vi "Microscope.TestLauncher.vi"() -> ()   [LabVIEW 2013]
doc: "JKI State Machine Objects (SMO) 1.0.0.5\nJKI - JKI\nCopyright (c) 2016, JKI"
uses:
  <vilib>/JKI/JKI SMO/SMO/SMO.lvclass
  Microscope.lvclass
  <vilib>/JKI/JKI SMO/SMO/Typedefs/SMOState --Enum.ctl
  <vilib>/Utility/error.llb/DialogType.ctl
  XYStage/Typedefs/(real)Coords--Cluster.ctl
  XYStage/XYStage.lvclass
  XYStage/Typedefs/PublicEvents--XYStage.UpdatedNamedPosition.ctl
  XYStage/Typedefs/PublicEvents--Cluster.ctl
  Camera/Typedefs/PublicEvents--Cluster.ctl
  Camera/Camera.lvclass
panel:
  in  "Settings":bool
  in  "Stop 2":bool caption="Stop"
  out "Camera model":string caption="CAMERA MODEL:"
  out "Image":picture
  out "Motion in Progress":bool
  out "Initialized":bool
  out "Well":string
  out "Position":string
  out "XYStage model":string caption="XY STAGE MODEL:"
  in  "Save Info":enum32{"Well Position", "Coordinates"}(radio)
  out "image path":path
  in  "Experiment":string
  in  "Save Images to Disk":bool
  out "Stage":picture
  in  "CaptureImmediately":bool
  in  "Coords":T1
  out "State":T2
  in  "CaptureAtPosition":bool
  out "error out":errorcluster
  # "MICROSCOPE CONTROLLER"
  # "Current Status"
  # "XY STAGE CONTROLLER"
  # "Current Address"
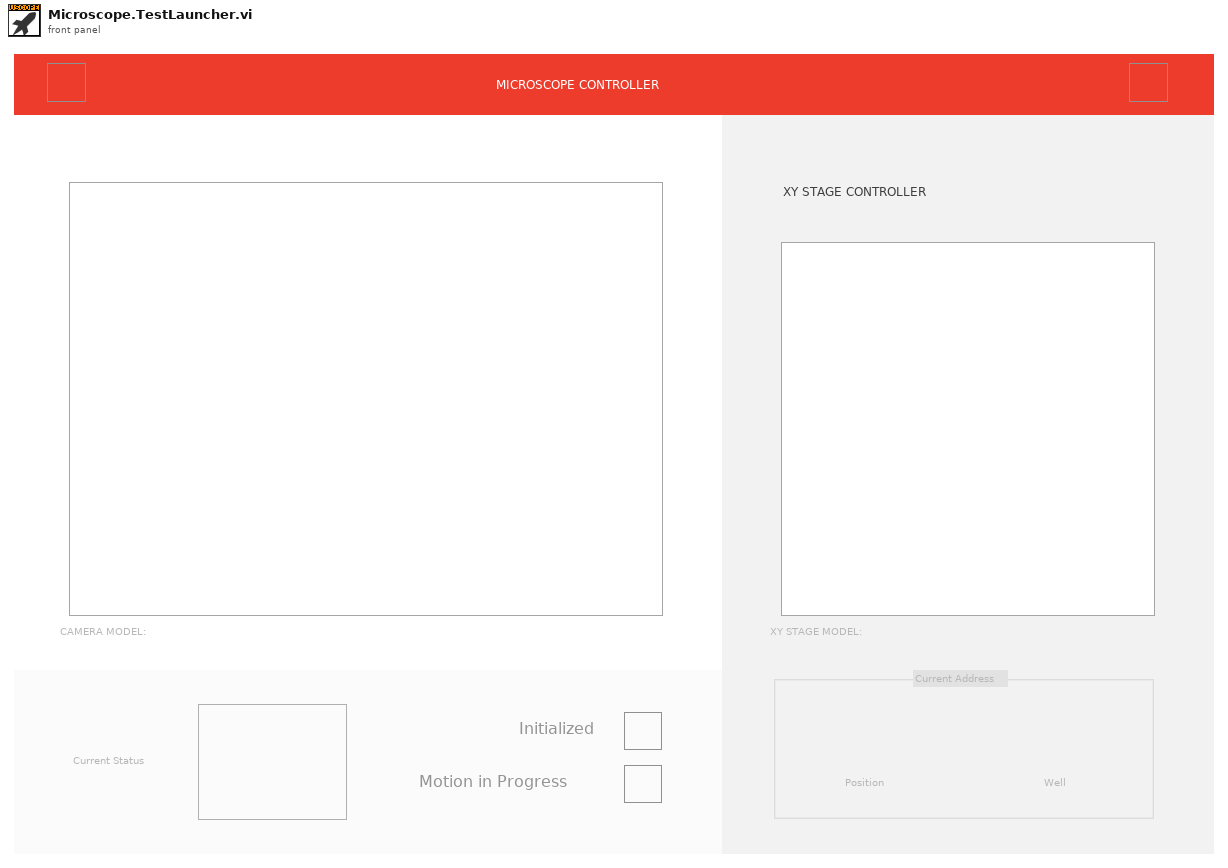
[diagram p1: front panel]
types:
  T1 = typedef "XYStage.lvclass/(real)Coords--Cluster.ctl" = cluster{"X":dbl, "Y":dbl}
  T2 = typedef "SMO.lvclass/SMOState --Enum.ctl" = enum16{"unknown", "Created", "Started", "Stopped"}
  T3 = cluster{"left":i16, "top":i16, "right":i16, "bottom":i16}
  T4 = typedef "Camera.lvclass/PublicEvents--Cluster.ctl" = cluster{"NewImage":refnum<user-event>, "ImageSaved":refnum<user-event>}
  T5 = typedef "XYStage.lvclass/PublicEvents--Cluster.ctl" = cluster{"MoveComplete":refnum<user-event>, "NewPosition":refnum<user-event>, "UpdatedNamedPosition":refnum<user-event>, "MoveStarted":refnum<user-event>}
  T6 = typedef "Microscope.lvclass/PublicEvents--Cluster.ctl" = cluster{"Value Changed":refnum<user-event>, "Initialized":refnum<user-event>}
  T7 = typedef "SMO.lvclass/Public Events.ctl" = cluster{"Error":refnum<user-event>, "State":refnum<user-event>}
  T8 = cluster{"Event Registration Refnum":refnum<event-registration>}
  T9 = typedef "imagedata.ctl" = cluster{"image type":i32, "image depth":i32, "image":u8[], "mask":u8[], "colors":u32[], "Rectangle":cluster{"left":i16, "top":i16, "right":i16, "bottom":i16}}
  T10 = typedef "LVMouseTypeDef.ctl" = cluster{"Mouse Position":cluster{"X":i32, "Y":i32}, "Mouse Modifiers":cluster{"Button Down":bool, "Shift Mod":bool, "Menu Mod":bool, "Option Mod":bool}}
  T11 = typedef "DialogType.ctl" = u16
  T12 = typedef "Microscope.lvclass/PublicEvents--Microscope.Initialized.ctl" = bool
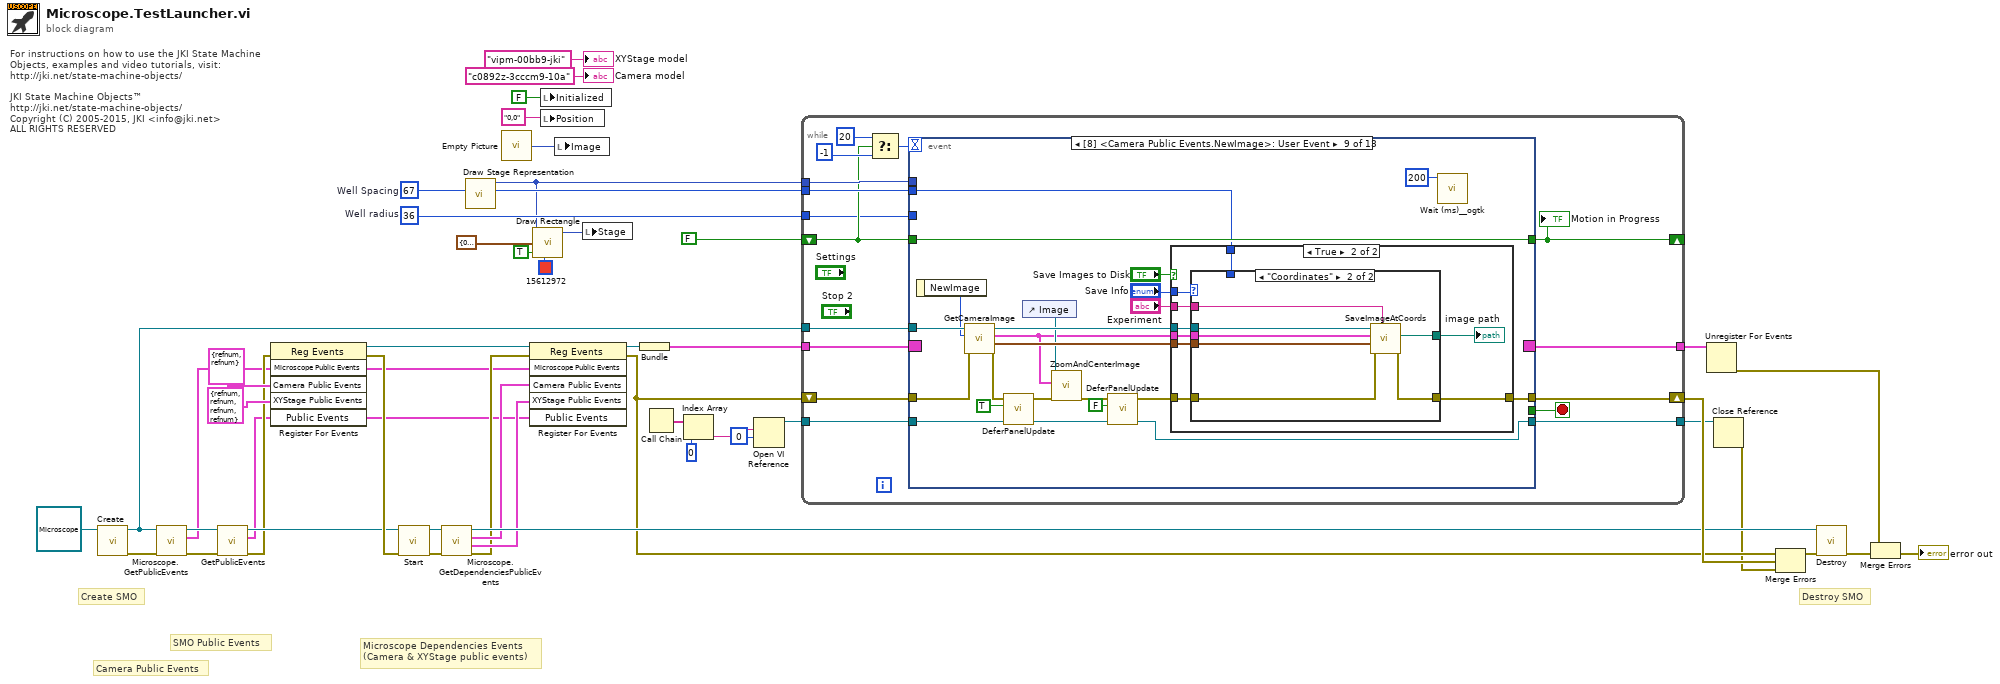
[diagram p0: block diagram]
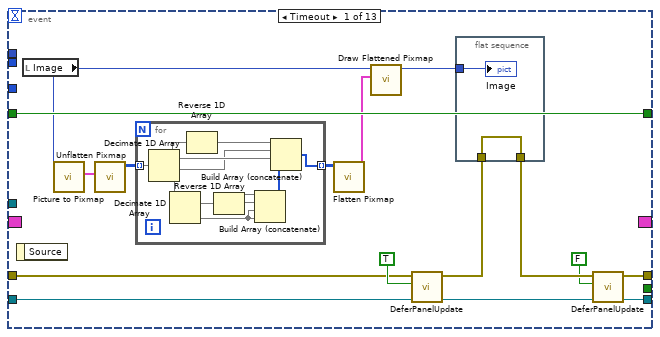
[diagram p2: hidden frame]
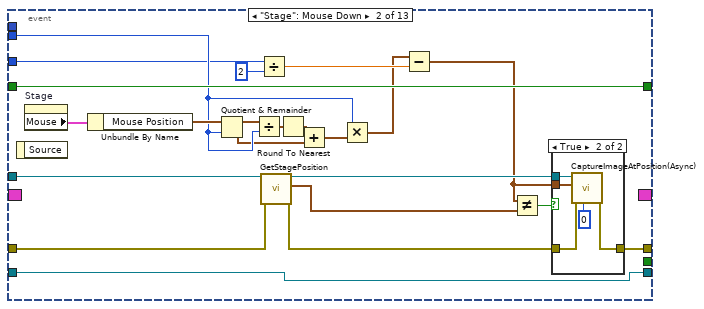
[diagram p3: hidden frame]
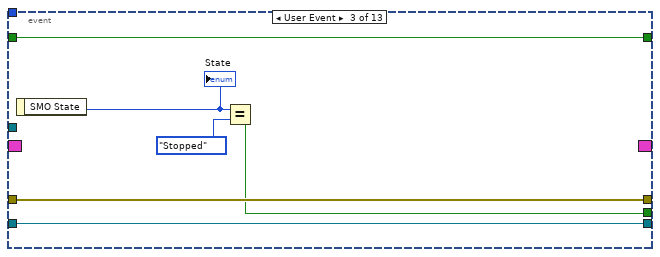
[diagram p5: hidden frame]
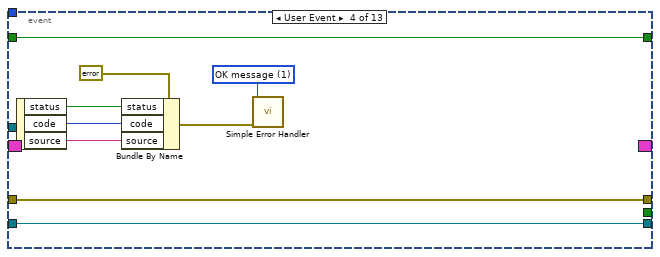
[diagram p6: hidden frame]
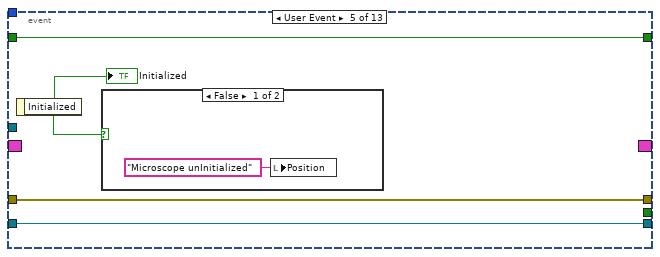
[diagram p7: hidden frame]
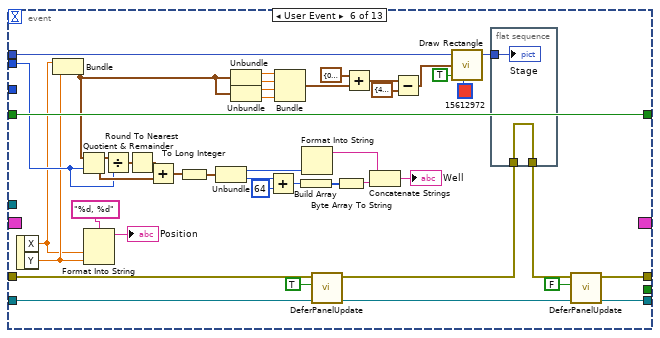
[diagram p9: hidden frame]
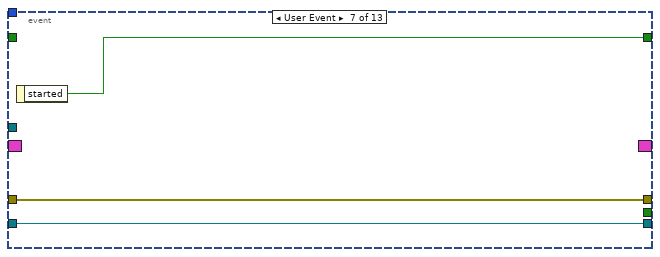
[diagram p10: hidden frame]
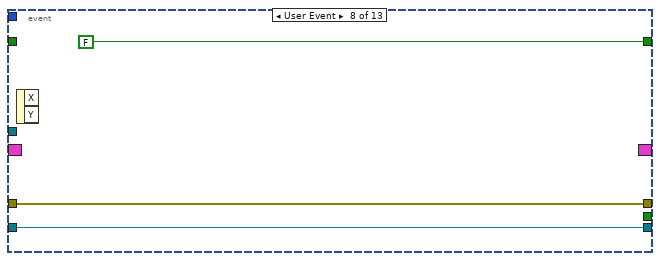
[diagram p11: hidden frame]
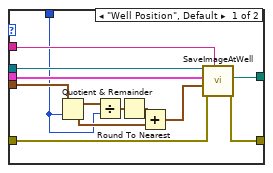
[diagram p13: hidden frame]
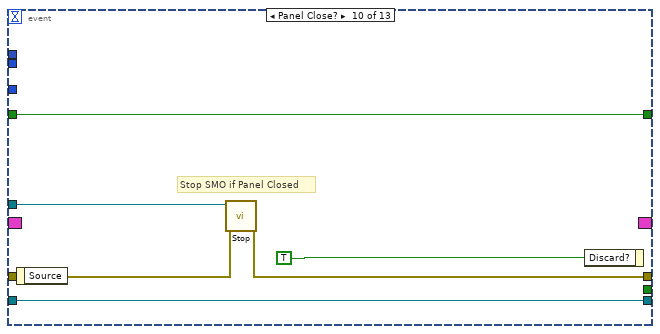
[diagram p14: hidden frame]
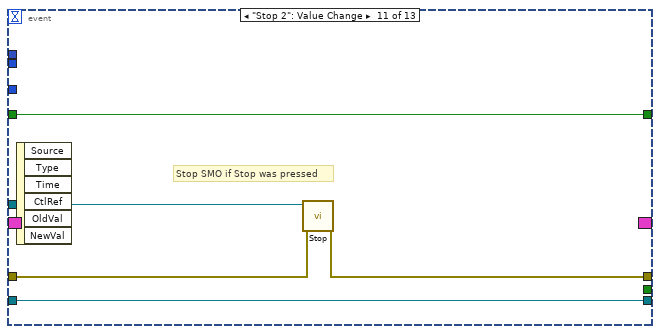
[diagram p15: hidden frame]
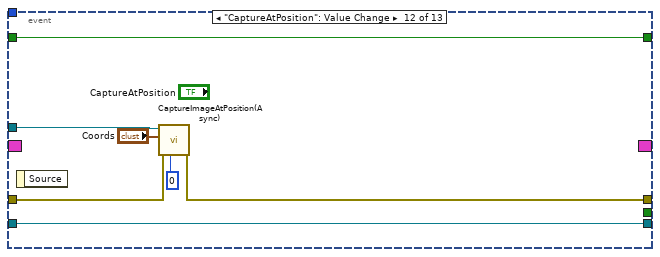
[diagram p16: hidden frame]
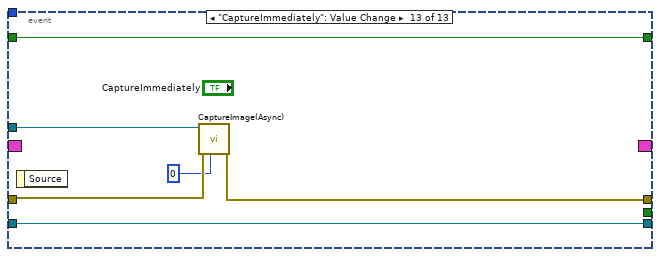
[diagram p17: hidden frame]
diagram:
  w15 = i16 36  # Well radius
  w3 = i16 67  # Well Spacing
  # "Microscope Dependencies Events\n(Camera & XYStage public events)"
  # "SMO Public Events"
  # "For instructions on how to use the JKI State Machine Objects, examples and video tutorials, visit:\nhttp://jki.net/state-machine-objects/\n\nJKI State Machine Objects™\nhttp://jki.net/state-machine-objects/\nCopyright (C) 2005-2015, JKI <info@jki.net>\nALL RIGHTS RESERVED"
  # "Camera Public Events"
  # "Destroy SMO"
  # "Create SMO"
  n1 = call <vilib>:"Create.vi"("SMO"=refnum<class "Microscope.lvclass"> refnum ("SMO.Template.lvclass")) -> ("error out"=w38:errorcluster, "SMO out"=w39:refnum<class "Microscope.lvclass">)  [unwired: 8 in, 1 out]
  n2 = call "Microscope.GetPublicEvents.vi"("error in (no error)"=w38, "Microscope"=w39) -> ("error out"=w41:errorcluster, "Microscope Public Events"=w19:T6, "Microscope out"=w42:refnum<class "Microscope.lvclass">)  [unwired: 7 in]
  n3 = call <vilib>:"GetPublicEvents.vi"("error in (no error)"=w41, "SMO"=w42) -> ("error out"=w29:errorcluster, "Public Events"=w18:T7, "SMO out"=w30:refnum<class "Microscope.lvclass">)  [unwired: 7 in]
  n4 = register-events(error in=w29, w19, T4 {"NewImage"=refnum, "ImageSaved"=refnum} ("Camera Public Events"), T5 {"MoveComplete"=refnum, "NewPosition"=refnum, "UpdatedNamedPosition"=refnum, "MoveStarted"=refnum} ("XYStage Public Events"), w18) -> (reference out=w25:refnum<event-registration>, error out=w37:errorcluster)  [unwired: 1 in]
  n5 = call <vilib>:"Start.vi"("error in (no error)"=w37, "SMO"=w30) -> ("error out"=w26:errorcluster, "SMO out"=w28:refnum<class "Microscope.lvclass">)  [unwired: 8 in]
  n6 = call "Microscope.GetDependenciesPublicEvents.vi"("error in (no error)"=w26, "Microscope"=w28) -> ("error out"=w21:errorcluster, "XYStage Public Events"=w22:T5, "Camera Public Events"=w23:T4, "Microscope out"=w27:refnum<class "Microscope.lvclass">)  [unwired: 6 in]
  n7 = call "Draw Stage Representation.vi"("Well Spacing"=w3) -> ("Well Spacing out"=w2:i16, "new picture"=w1:picture)  [unwired: 9 in]
  n8 = call "Empty Picture"() -> ("empty picture"=w33:picture)
  n9 = register-events(reference=w25, error in=w21, w19, w23, w22, w18) -> (reference out=w24:refnum<event-registration>, error out=w20:errorcluster)
  n10 = call <vilib>:"Draw Rectangle.vi"("picture"=w1, "rect"=T3 {"left"=0, "top"=0, "right"=6, "bottom"=6}, "fill?(F)"=TRUE, "color(black)"=u32 15612972) -> ("new picture"=w11:picture)  [unwired: 5 in]
  n11 = local write "Initialized"(FALSE ("Initialized")) -> ()
  n12 = local write "Position"("0,0" ("Position")) -> ()
  n13 = local write "Image"(w33) -> ()
  n14 = local write "Stage"(w11) -> ()
  n15 = Bundle("Event Registration Refnum"=w24) -> (w48:T8)  [unwired: 1 in]
  n16 = Call Chain() -> (call chain=w7:string[])
  n17 = Index Array(array=w7, index=0 ("Index")) -> (element=w9:string)
  n18 = Open VI Reference(vi path=w9, options=0) -> (vi reference=w6:refnum<vi>)  [unwired: 4 in, 1 out]
  n19 = while {
    shift-right: [w64] -> w47
    shift-left: w20 -> [w63]
    tunnel: w48 -> [w62]
    tunnel: [w61] -> w49
    tunnel: w39 -> [w60]
    shift-right: [w59] -> _
    shift-left: FALSE -> [w54]
    tunnel: w1 -> [w58]
    tunnel: w2 -> [w57]
    tunnel: w15 -> [w52]
    tunnel: w6 -> [w51]
    tunnel: [w50] -> w5
    stop <- w65 stop-if-true
    n20 = Select(t=20, s=w54, f=-1) -> (s? t:f=w55:i32)
    n21 = event shown="[8] <Camera Public Events.NewImage>: User Event" {
      selector: w62 -> [_ _ _ _ _ _ _ _ _ _ _ _ _]
      dyn-events: [_ _ _ _ _ _ _ _ _ _ _ _ _] -> w61
      timeout: w55 -> [_ _ _ _ _ _ _ _ _ _ _ _ _]
      tunnel: [_ _ w125 _ _ _ _ _ _ _ _ _ _] -> w65
      tunnel: w60 -> [_ w106 _ _ _ _ _ _ w216 w252 w257 w263 w270]
      tunnel: [w73 w114 w128 w137 w141 w145 w190 w193 w211 w251 w256 w259 w268] -> w64
      tunnel: w63 -> [w76 w104 w128 w137 w141 w150 w190 w193 w214 w250 w255 w261 w269]
      tunnel: [w81 w116 w124 w136 w139 w183 w189 FALSE w213 w248 w254 w264 w266] -> w59
      tunnel: w54 -> [w81 w116 w124 w136 w139 w183 _ _ w213 w248 w254 w264 w266]
      tunnel: w58 -> [_ _ _ _ _ w168 _ _ _ _ _ _ _]
      tunnel: w57 -> [_ w112 _ _ _ w178 _ _ w206 _ _ _ _]
      tunnel: w52 -> [_ w101 _ _ _ _ _ _ _ _ _ _ _]
      tunnel: w51 -> [w74 w95 w123 w129 w138 w149 w188 w191 w202 w247 w253 w258 w265]
      tunnel: [w72 w95 w123 w129 w138 w143 w188 w191 w198 w247 w253 w258 w265] -> w50
      event Timeout {
        n22 = event-data() -> ()  [unwired: 1 in, 1 out]
        n23 = local read "Image"() -> (w68:picture)
        n24 = call <vilib>:"Picture to Pixmap.vi"("picture"=w68) -> ("image data"=w80:T9)  [unwired: 9 in, 1 out]
        n25 = call <vilib>:"Unflatten Pixmap.vi"("image data"=w80) -> ("24-bit pixmap"=w79:u32[][])  [unwired: 4 in, 6 out]
        n26 = for {
          tunnel: w79 -> [w94] mode=indexing
          tunnel: [w90] -> w78 mode=indexing
          n27 = Decimate 1D Array(w94) -> (w93:u32[], w92:u32[], w91:u32[], w89:u32[])
          n28 = Decimate 1D Array(w89) -> (w88:u32[], w85:u32[])  [unwired: 2 out]
          n29 = Reverse 1D Array(array=w93) -> (reversed array=w87:u32[])
          n30 = Reverse 1D Array(array=w88) -> (reversed array=w86:u32[])
          n31 = Build Array (concatenate)(w86, w86, w85, w85) -> (w84:u32[])
          n32 = Build Array (concatenate)(w87, w91, w92, w84) -> (w90:u32[])
        }
        n33 = call <vilib>:"Flatten Pixmap.vi"("24-bit pixmap"=w78) -> ("image data"=w67:T9)  [unwired: 10 in]
        n34 = call <vilib>:"Draw Flattened Pixmap.vi"("image data"=w67, "picture"=w68) -> ("new picture"=w66:picture)  [unwired: 7 in]
        n35 = call "DeferPanelUpdate.vi"("VI in"=w74, "defer panel updates"=TRUE, "error in (no error)"=w76) -> ("VI out"=w71:refnum<vi>, "error out"=w75:errorcluster)  [unwired: 7 in]
        n36 = flat-sequence {
          tunnel: w66 -> [w83]
          tunnel: [w82] -> w70
          tunnel: w75 -> [w82]
          frame #0 {
            "Image" <- w83
          }
        }
        n37 = call "DeferPanelUpdate.vi"("VI in"=w71, "defer panel updates"=FALSE, "error in (no error)"=w70) -> ("VI out"=w72:refnum<vi>, "error out"=w73:errorcluster)  [unwired: 7 in]
      }
      event "Stage": Mouse Down {
        n38 = event-data() -> ()  [unwired: 1 in, 1 out]
        n39 = property on="Stage" class="Pict"() -> ("Mouse"=w115:T10)  [unwired: 2 in, 2 out]
        n40 = Unbundle By Name(w115) -> ("Mouse Position"=w113:cluster{"X":i32, "Y":i32})
        n41 = Quotient & Remainder(x=w113, y=w112) -> (x-y*floor(x/y)=w110:cluster{"X":i32, "Y":i32}, floor(x/y)=w108:cluster{"X":i32, "Y":i32})
        n42 = Divide(x=w110, y=w112) -> (x/y=w111:cluster{"X":dbl, "Y":dbl})
        n43 = Divide(x=w101, y=i16 2) -> (x/y=w99:dbl)
        n44 = call "GetStagePosition.vi"("error in (no error)"=w104, "Microscope"=w106) -> ("error out"=w103:errorcluster, "Coords"=w102:T1, "Microscope out"=w105:refnum<class "Microscope.lvclass">)  [unwired: 7 in]
        n45 = Round To Nearest(number=w111) -> (nearest integer value=w109:cluster{"X":dbl, "Y":dbl})
        n46 = Add(x=w109, y=w108) -> (x+y=w98:cluster{"X":dbl, "Y":dbl})
        n47 = Multiply(x=w112, y=w98) -> (x*y=w97:cluster{"X":dbl, "Y":dbl})
        n48 = Subtract(x=w97, y=w99) -> (x-y=w96:cluster{"X":dbl, "Y":dbl})
        n49 = Not Equal?(x=w96, y=w102) -> (x != y?=w107:bool)
        n50 = case shown="True" w107 {
          tunnel: w105 -> [_ w122]
          tunnel: w103 -> [w117 w120]
          tunnel: [w117 w119] -> w114
          tunnel: w96 -> [_ w121]
          frame False {
          }
          frame True {
            n51 = call "CaptureImageAtPosition(Async).vi"("timeout in ms (5000)"=0, "error in (no error)"=w120, "Coords"=w121, "Microscope"=w122) -> ("error out"=w119:errorcluster)  [unwired: 5 in, 2 out]
          }
        }
      }
      event User Event {
        n52 = event-data() -> ("SMO State"=w127:T2)  [unwired: 1 in]
        "State" <- w127
        n53 = Equal?(x=w127, y=SMOState_--Enum."Stopped") -> (x = y?=w125:bool)
      }
      event User Event {
        w133 = T11 1 items=["no dialog", "OK message", "continue or stop message", "OK message + warnings", "continue/stop + warnings"] ("type of dialog (OK msg:1)")
        n54 = event-data() -> ("status"=w132:bool, "code"=w131:i32, "source"=w130:string)  [unwired: 1 in]
        n55 = Bundle By Name(cluster=errorcluster {"status"=FALSE, "code"=0, "source"=""} ("error out"), "status"=w132, "code"=w131, "source"=w130) -> (w134:errorcluster)
        n56 = call <vilib>:"Simple Error Handler.vi"("type of dialog (OK msg:1)"=w133, "error in (no error)"=w134) -> ()  [unwired: 3 in, 5 out]
      }
      event User Event {
        n57 = event-data() -> ("Initialized"=w140:T12)  [unwired: 1 in]
        "Initialized" <- w140
        n58 = case shown="False" w140 {
          frame False {
            n59 = local write "Position"("Microscope unInitialized" ("Position")) -> ()
          }
          frame True {
          }
        }
      }
      event User Event {
        n60 = event-data() -> ("X"=w161:dbl, "Y"=w162:dbl)  [unwired: 1 in]
        n61 = Bundle("X"=w161, "Y"=w162) -> (w159:cluster{"X":dbl, "Y":dbl})  [unwired: 1 in]
        n62 = Quotient & Remainder(x=w159, y=w178) -> (x-y*floor(x/y)=w181:cluster{"X":dbl, "Y":dbl}, floor(x/y)=w179:cluster{"X":dbl, "Y":dbl})
        n63 = Format Into String(format string="%d, %d", w161, w162) -> (resulting string=→"Position":string)  [unwired: 2 in, 1 out]
        n64 = Divide(x=w181, y=w178) -> (x/y=w182:cluster{"X":dbl, "Y":dbl})
        n65 = Round To Nearest(number=w182) -> (nearest integer value=w180:cluster{"X":dbl, "Y":dbl})
        n66 = Add(x=w180, y=w179) -> (x+y=w177:cluster{"X":dbl, "Y":dbl})
        n67 = To Long Integer(number=w177) -> (32bit integer=w176:cluster{"X":i32, "Y":i32})
        n68 = Unbundle(w176) -> ("X"=w171:i32, "Y"=w175:i32)
        n69 = Unbundle(w159) -> ("X"=w158:dbl, "Y"=w157:dbl)
        n70 = Unbundle(w159) -> ("X"=w160:dbl, "Y"=w156:dbl)
        n71 = Add(x=w175, y=64 ("x")) -> (x+y=w173:i32)
        n72 = Bundle("X"=w158, "Y"=w157, "X"=w160, "Y"=w156) -> (w164:cluster{"X":dbl, "Y":dbl, "X":dbl, "Y":dbl})  [unwired: 1 in]
        n73 = Build Array(w173) -> (w174:i32[])
        n74 = Format Into String(w171) -> (resulting string=w152:string)  [unwired: 3 in, 1 out]
        n75 = call "DeferPanelUpdate.vi"("VI in"=w149, "defer panel updates"=TRUE, "error in (no error)"=w150) -> ("VI out"=w144:refnum<vi>, "error out"=w148:errorcluster)  [unwired: 7 in]
        n76 = Byte Array To String(unsigned byte array=w174) -> (string=w170:string)
        n77 = Add(x=T3 {"left"=0, "top"=0, "right"=13, "bottom"=13} ("rect"), y=w164) -> (x+y=w155:cluster{dbl, dbl, dbl, dbl})
        n78 = Concatenate Strings(w152, w170) -> (→"Well":string)
        n79 = Subtract(x=w155, y=cluster{dbl, dbl, dbl, dbl} {4.0, 3.0, 4.0, 3.0}) -> (x-y=w154:cluster{dbl, dbl, dbl, dbl})
        n80 = call <vilib>:"Draw Rectangle.vi"("picture"=w168, "rect"=w154, "fill?(F)"=TRUE, "color(black)"=u32 15612972) -> ("new picture"=w165:picture)  [unwired: 5 in]
        n81 = flat-sequence {
          tunnel: w165 -> [w187]
          tunnel: [w186] -> w146
          tunnel: w148 -> [w186]
          frame #0 {
            "Stage" <- w187
          }
        }
        n82 = call "DeferPanelUpdate.vi"("VI in"=w144, "defer panel updates"=FALSE, "error in (no error)"=w146) -> ("VI out"=w143:refnum<vi>, "error out"=w145:errorcluster)  [unwired: 7 in]
      }
      event User Event {
        n83 = event-data() -> ("started"=w189:bool)  [unwired: 1 in]
      }
      event User Event {
        n84 = event-data() -> ()  [unwired: 1 in, 2 out]
      }
      event User Event {
        n85 = event-data() -> ("NewImage"=w215:i32)  [unwired: 1 in]
        n86 = call "GetCameraImage.vi"("error in (no error)"=w214, "Get Image (-1: latest)"=w215, "Microscope"=w216) -> ("error out"=w204:errorcluster, "Coords"=w210:T1, "image data"=w194:T9, "Microscope out"=w212:refnum<class "Microscope.lvclass">)  [unwired: 5 in]
        n87 = call "DeferPanelUpdate.vi"("VI in"=w202, "defer panel updates"=TRUE, "error in (no error)"=w204) -> ("VI out"=w199:refnum<vi>, "error out"=w197:errorcluster)  [unwired: 7 in]
        n88 = control-ref of="Image"() -> (w195:refnum<vi>)
        n89 = call "ZoomAndCenterImage.vi"("error in (no error)"=w197, "image data"=w194, "Picture Ref"=w195) -> ("error out"=w196:errorcluster)  [unwired: 8 in]
        n90 = call "DeferPanelUpdate.vi"("VI in"=w199, "defer panel updates"=FALSE, "error in (no error)"=w196) -> ("VI out"=w198:refnum<vi>, "error out"=w201:errorcluster)  [unwired: 7 in]
        n91 = case shown="True" "Save Images to Disk" {
          tunnel: w212 -> [_ w226]
          tunnel: w201 -> [w217 w225]
          tunnel: [w217 w224] -> w211
          tunnel: w194 -> [_ w223]
          tunnel: w210 -> [_ w222]
          tunnel: "Experiment" -> [_ w220]
          tunnel: "Save Info" -> [_ w219]
          tunnel: w206 -> [_ w218]
          frame False {
          }
          frame True {
            n92 = case shown="\"Coordinates\"" w219 {
              tunnel: w226 -> [w239 w246]
              tunnel: w225 -> [w236 w245]
              tunnel: [w235 w244] -> w224
              tunnel: w223 -> [w238 w243]
              tunnel: w222 -> [w230 w242]
              tunnel: [w227 w241] -> w221
              tunnel: w220 -> [w237 w240]
              tunnel: w218 -> [w228 _]
              frame "Well Position", Default {
                n93 = Quotient & Remainder(x=w230, y=w228) -> (x-y*floor(x/y)=w233:T1, floor(x/y)=w231:T1)
                n94 = Divide(x=w233, y=w228) -> (x/y=w234:T1)
                n95 = Round To Nearest(number=w234) -> (nearest integer value=w232:T1)
                n96 = Add(x=w232, y=w231) -> (x+y=w229:T1)
                n97 = call "SaveImageAtWell.vi"("namespace"=w237, "error in (no error)"=w236, "Well"=w229, "image data"=w238, "Microscope"=w239) -> ("error out"=w235:errorcluster, "image path"=w227:path)  [unwired: 4 in, 1 out]
              }
              frame "Coordinates" {
                n98 = call "SaveImageAtCoords.vi"("namespace"=w240, "error in (no error)"=w245, "Coords"=w242, "image data"=w243, "Microscope"=w246) -> ("error out"=w244:errorcluster, "image path"=w241:path)  [unwired: 4 in, 1 out]
              }
            }
            "image path" <- w221
          }
        }
        n99 = call "Wait (ms)__ogtk.vi"("milliseconds to wait"=u32 200) -> ()  [unwired: 9 in, 2 out]
      }
      event Panel Close? {
        # "Stop SMO if Panel Closed"
        n100 = event-data() -> ()  [unwired: 1 in, 1 out]
        n101 = call <vilib>:"Stop.vi"("error in (no error)"=w250, "SMO"=w252) -> ("error out"=w251:errorcluster)  [unwired: 8 in, 1 out]
        n102 = event-data("Discard?"=TRUE ("OK")) -> ()  [unwired: 1 in, 1 out]
      }
      event "Stop 2": Value Change {
        # "Stop SMO if Stop was pressed"
        n103 = event-data() -> ()  [unwired: 1 in, 6 out]
        n104 = call <vilib>:"Stop.vi"("error in (no error)"=w255, "SMO"=w257) -> ("error out"=w256:errorcluster)  [unwired: 8 in, 1 out]
      }
      event "CaptureAtPosition": Value Change {
        n105 = event-data() -> ()  [unwired: 1 in, 1 out]
        n106 = call "CaptureImageAtPosition(Async).vi"("timeout in ms (5000)"=0, "error in (no error)"=w261, "Coords"="Coords", "Microscope"=w263) -> ("error out"=w259:errorcluster)  [unwired: 5 in, 2 out]
      }
      event "CaptureImmediately": Value Change {
        n107 = event-data() -> ()  [unwired: 1 in, 1 out]
        n108 = call "CaptureImage(Async).vi"("timeout in ms (5000)"=0, "error in (no error)"=w269, "Microscope"=w270) -> ("error out"=w268:errorcluster)  [unwired: 6 in, 2 out]
      }
    }
    "Motion in Progress" <- w59
  }
  n109 = Unregister For Events(event registration refnum=w49) -> (error out=w46:errorcluster)  [unwired: 1 in]
  n110 = Close Reference(reference=w5) -> (error out=w4:errorcluster)  [unwired: 1 in]
  n111 = Merge Errors(w20, w47, w4) -> (w40:errorcluster)
  n112 = call <vilib>:"Destroy.vi"("error in (no error)"=w40, "SMO"=w27) -> ("error out"=w44:errorcluster)  [unwired: 9 in]
  n113 = Merge Errors(w46, w44) -> (→"error out":errorcluster)
  "XYStage model" <- "vipm-00bb9-jki" ("XYStage model")
  "Camera model" <- "c0892z-3cccm9-10a" ("Camera model")
